vi "Get Module Object.vi"(8 "error in (no error)":errorcluster, 9 "Assembly Tray Position":i32, 10 "Assembly Tray Region":i32, 11 "Assembly Tray Number":i32) -> (0 "error out":errorcluster, 3 "Module.lvclass":refnum<class "Module.lvclass">)   [LabVIEW 2016, in "Module.lvclass"]
uses:
  Module.lvclass
  Module.lvclass/Module.ctl
  Workspace/Fixture.lvclass
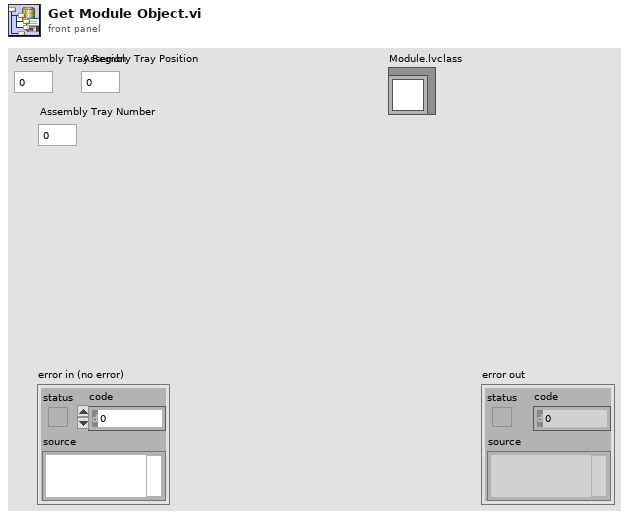
[diagram p1: front panel]
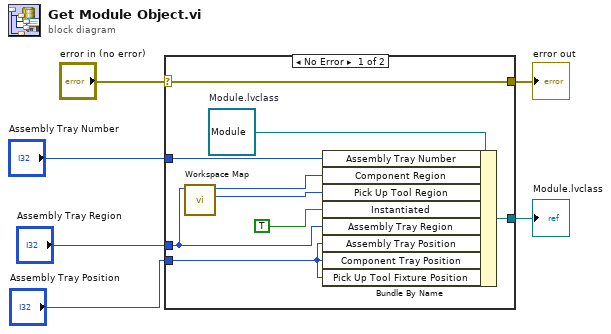
[diagram p0: block diagram]
diagram:
  n1 = case shown="No Error" "error in (no error)" {
    selector: "error in (no error)" -> [w15 w16]
    tunnel: [w15 w16] -> w5
    tunnel: "Assembly Tray Number" -> [w9 _]
    tunnel: "Assembly Tray Region" -> [w8 _]
    tunnel: [w13 _] -> w2
    tunnel: "Assembly Tray Position" -> [w7 _]
    frame No Error {
      w14 = refnum<class "Module.lvclass"> refnum  # Module.lvclass
      n2 = call "Workspace Map.vi"("Assembly Tray Region"=w8) -> ("Pick Up Tool Region"=w11:i32, "Component Tray Region"=w12:i32)  [unwired: 9 in]
      n3 = Bundle By Name(cluster=w14, "Assembly Tray Number"=w9, "Component Region"=w12, "Pick Up Tool Region"=w11, "Instantiated"=TRUE, "Assembly Tray Region"=w8, "Assembly Tray Position"=w7, "Component Tray Position"=w7, "Pick Up Tool Fixture Position"=w7) -> (w13:refnum<class "Module.lvclass">)
    }
    frame Error {
    }
  }
  "error out" <- w5
  "Module.lvclass" <- w2
